vi "Refactor Object for File Rename.vi"(8 "error in (no error)":errorcluster, 10 "rename data":T2, 11 "object reference in":refnum<vi>) -> (0 "error out":errorcluster, 1 "refactored dependency":bool, 2 "refactor result":T1, 3 "object reference out":refnum<vi>)   [LabVIEW 2020, in "MeasurementService Editor.lvlib"]
uses:
  MeasurementService Editor.lvlib
  Rename Refactor Data.ctl
  Rename Refactor Mapping Info.ctl
  Rename Refactor Result.ctl
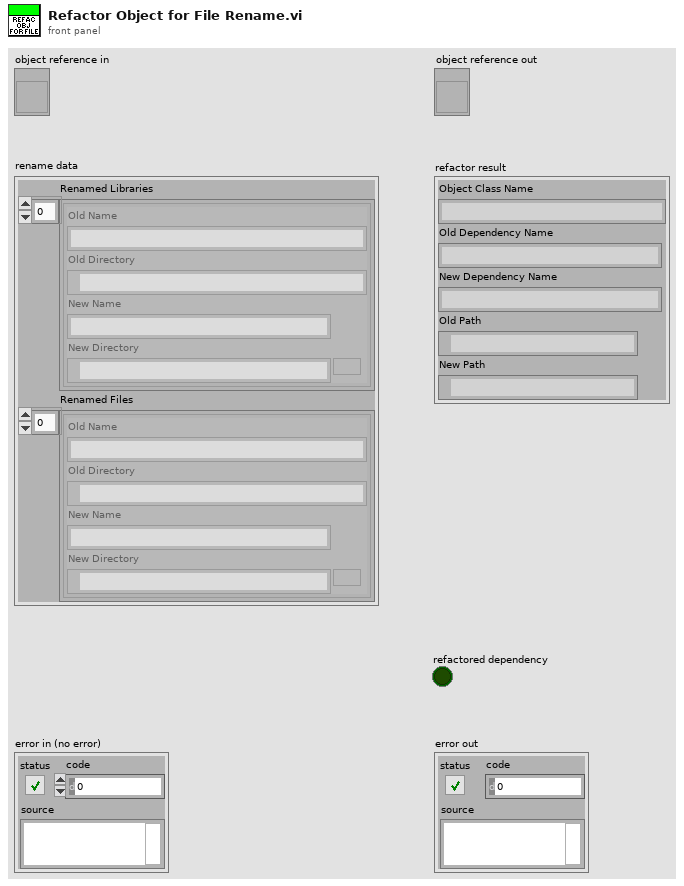
[diagram p1: front panel]
types:
  T1 = typedef "MeasurementService Editor.lvlib/Rename Refactor Result.ctl" = cluster{"Object Class Name":string, "Old Dependency Name":string, "New Dependency Name":string, "Old Path":path, "New Path":path}
  T2 = typedef "MeasurementService Editor.lvlib/Rename Refactor Data.ctl" = cluster{"Renamed Libraries":T3[], "Renamed Files":T3[]}
  T3 = typedef "MeasurementService Editor.lvlib/Rename Refactor Mapping Info.ctl" = cluster{"Old Name":string, "Old Directory":path, "New Name":string, "New Directory":path}
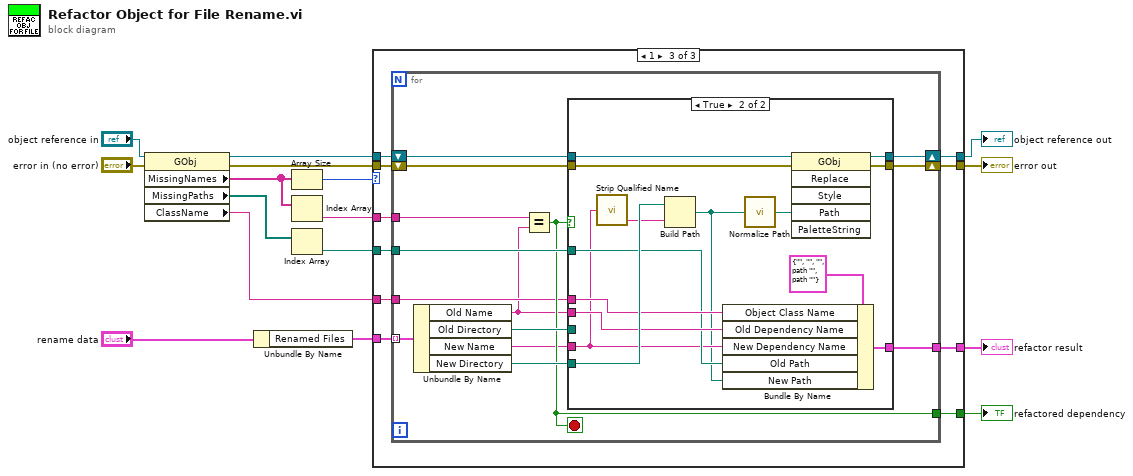
[diagram p0: block diagram]
diagram:
  n1 = property class="GObj"(reference="object reference in", error in="error in (no error)") -> (reference out=w12:refnum<vi>, error out=w11:errorcluster, "MissingNames"=w10:string[], "MissingPaths"=w6:path[], "ClassName"=w7:string)
  n2 = Unbundle By Name("rename data") -> ("Renamed Files"=w5:T3[])
  n3 = Array Size(array=w10) -> (size(s)=w8:i32)
  n4 = Index Array(array=w10) -> (element=w9:string)  [unwired: 1 in]
  n5 = Index Array(array=w6) -> (element=w4:path)  [unwired: 1 in]
  n6 = case shown="1" w8 {
    tunnel: w12 -> [w17 w19 w30]
    tunnel: w11 -> [w18 w20 w29]
    tunnel: w9 -> [_ _ w27]
    tunnel: [w18 w20 w23] -> w16
    tunnel: [w17 w19 w24] -> w3
    tunnel: w7 -> [_ _ w25]
    tunnel: w4 -> [_ _ w26]
    tunnel: w5 -> [_ _ w28]
    tunnel: [_ _ w22] -> w1
    tunnel: [_ _ w21] -> w2
    frame 0 {
    }
    frame Default {
      # "Maybe generate warning?"
    }
    frame 1 {
      n7 = for {
        shift-right: [w39] -> w23
        shift-left: w29 -> [w41]
        shift-right: [w40] -> w24
        shift-left: w30 -> [w42]
        tunnel: w28 -> [w44] mode=indexing
        tunnel: w27 -> [w43]
        tunnel: w26 -> [w37]
        tunnel: [w35] -> w22
        tunnel: w25 -> [w34]
        tunnel: [w31] -> w21
        stop <- w35 stop-if-true
        n8 = Unbundle By Name(w44) -> ("Old Name"=w33:string, "Old Directory"=w38:path, "New Name"=w32:string, "New Directory"=w36:path)
        n9 = Equal?(x=w43, y=w33) -> (x = y?=w35:bool)
        n10 = case shown="True" w35 {
          tunnel: w42 -> [w46 w57]
          tunnel: w41 -> [w45 w51]
          tunnel: [w46 w58] -> w40
          tunnel: [w45 w59] -> w39
          tunnel: w38 -> [_ _]
          tunnel: w37 -> [_ w53]
          tunnel: w36 -> [_ w60]
          tunnel: w34 -> [_ w55]
          tunnel: w33 -> [_ w54]
          tunnel: w32 -> [_ w50]
          tunnel: [_ w52] -> w31
          frame False {
          }
          frame True {
            n11 = call "Strip Qualified Name.vi"("name"=w50) -> ("stripped name"=w49:string)  [unwired: 5 in, 1 out]
            n12 = Build Path(base path=w60, name or relative path=w49) -> (appended path=w48:path)
            n13 = Bundle By Name(cluster=T1 {"Object Class Name"="", "Old Dependency Name"="", "New Dependency Name"="", "Old Path"=path "", "New Path"=path ""} ("Rename Refactor Result"), "Object Class Name"=w55, "Old Dependency Name"=w54, "New Dependency Name"=w50, "Old Path"=w53, "New Path"=w48) -> (w52:T1)
            n14 = call "Normalize Path.vi"("path"=w48) -> ("normalized path"=w47:path)
            n15 = invoke class="GObj" method="Replace"(reference=w57, error in=w51, "Path"=w47) -> (reference out=w58:refnum<vi>, error out=w59:errorcluster)  [unwired: 3 in, 4 out]
          }
        }
      }
    }
  }
  "error out" <- w16
  "object reference out" <- w3
  "refactor result" <- w2
  "refactored dependency" <- w1
